vi "Rename Line.vi"(8 "error in":errorcluster, 9 "new name":string, 10 "old name":string, 11 "module configuration in":refnum<class "tag bus configurable plugin module configuration.lvclass">) -> (0 "error out":errorcluster, 3 "module configuration out":refnum<class "tag bus configurable plugin module configuration.lvclass">)   [LabVIEW 2013]
uses:
  <vilib>/NI/Tag Bus/tag/tag descriptor.lvclass
  tag bus configurable plugin module configuration.lvclass
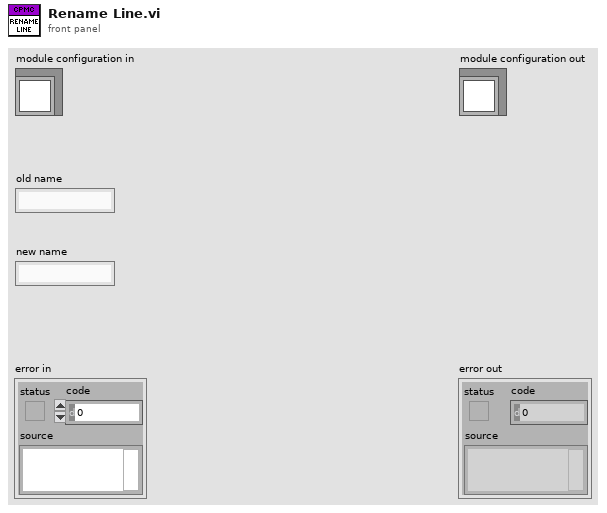
[diagram p1: front panel]
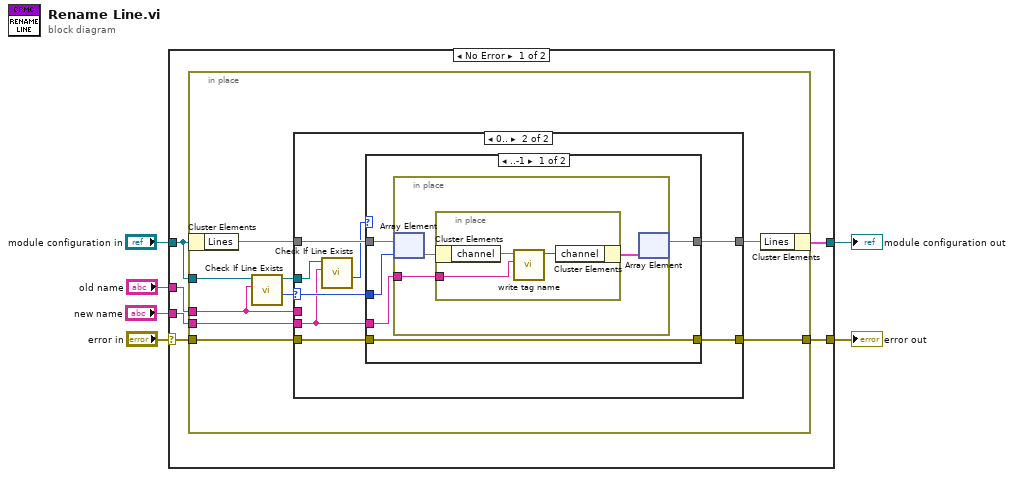
[diagram p0: block diagram]
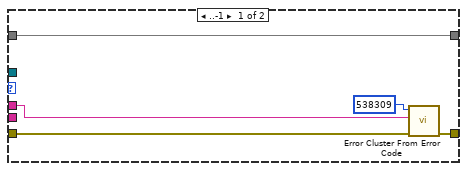
[diagram p2: hidden frame]
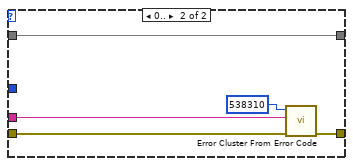
[diagram p3: hidden frame]
diagram:
  n1 = case shown="No Error" "error in" {
    selector: "error in" -> [w8 w52]
    tunnel: "new name" -> [w12 _]
    tunnel: "module configuration in" -> [w7 w51]
    tunnel: [w11 w51] -> w4
    tunnel: [w10 w52] -> w3
    tunnel: "old name" -> [w9 _]
    frame No Error {
      n2 = in-place {
        in-place-border: w9 -> [w15]
        in-place-border: w12 -> [w17]
        in-place-border: [w20] -> w10
        in-place-border: w8 -> [w18]
        in-place-border: w7 -> [w16]
        n3 = in-place-cluster #1(w7) -> ("Lines"=w21)
        n4 = call-dynamic "Check If Line Exists.vi"("name to locate"=w15, "tag bus configurable plugin module configuration in"=w16) -> ("index"=w14:i32, "tag bus configurable plugin module configuration out"=w13:refnum<class "tag bus configurable plugin module configuration.lvclass">)  [unwired: 6 in, 2 out]
        n5 = case shown="0.." w14 {
          selector: w14 -> [_ w30]
          tunnel: w21 -> [w23 w33]
          tunnel: w15 -> [w25 _]
          tunnel: [w24 w31] -> w20
          tunnel: [w23 w34] -> w19
          tunnel: w18 -> [w22 w32]
          tunnel: w17 -> [_ w28]
          tunnel: w13 -> [_ w29]
          frame ..-1 {
            n6 = call <vilib>:"Error Cluster From Error Code.vi"("error in (no error)"=w22, "error message (\"\")"=w25, "error code (0)"=538309) -> ("error out"=w24:errorcluster)  [unwired: 6 in]
          }
          frame 0.. {
            n7 = call-dynamic "Check If Line Exists.vi"("name to locate"=w28, "tag bus configurable plugin module configuration in"=w29) -> ("index"=w27:i32)  [unwired: 6 in, 3 out]
            n8 = case shown="..-1" w27 {
              tunnel: [w39 w50] -> w34
              tunnel: w30 -> [w38 _]
              tunnel: w33 -> [w37 w50]
              tunnel: w28 -> [w36 w46]
              tunnel: w32 -> [w35 w48]
              tunnel: [w35 w49] -> w31
              frame ..-1 {
                n9 = in-place {
                  in-place-border: w36 -> [w42]
                  n10 = in-place-array #2(w37, w38) -> (w41)
                  n11 = in-place {
                    in-place-border: w42 -> [w45]
                    n12 = in-place-cluster #3(w41) -> ("channel"=w44)
                    n13 = call <vilib>:"write tag name.vi"("name"=w45, "system tag in"=w44) -> ("system tag out"=w43:refnum<class "tag descriptor.lvclass">)  [unwired: 8 in, 1 out]
                    n14 = in-place-cluster #3("channel"=w43) -> (w40:cluster{})
                  }
                  n15 = in-place-array #2(w40) -> (w39)  [unwired: 1 out]
                }
              }
              frame 0.. {
                n16 = call <vilib>:"Error Cluster From Error Code.vi"("error in (no error)"=w48, "error message (\"\")"=w46, "error code (0)"=538310) -> ("error out"=w49:errorcluster)  [unwired: 6 in]
              }
            }
          }
        }
        n17 = in-place-cluster #1("Lines"=w19) -> (w11:cluster{})
      }
    }
    frame Error {
    }
  }
  "error out" <- w3
  "module configuration out" <- w4
